vi "prase 4 parameter numeric.vi"(0 "value":string) -> (1 "Settings.Gain.Min 4":dbl, 2 "Settings.Gain.Min 3":dbl, 3 "Settings.Gain.Min 2":dbl, 4 "Settings.Gain.Min":dbl)   [LabVIEW 2011, in "MoveDataFile.lvclass"]
uses:
  MoveDataFile.lvclass
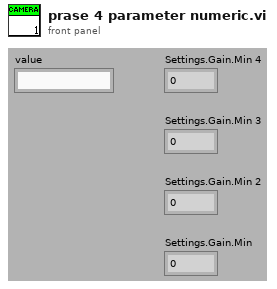
[diagram p1: front panel]
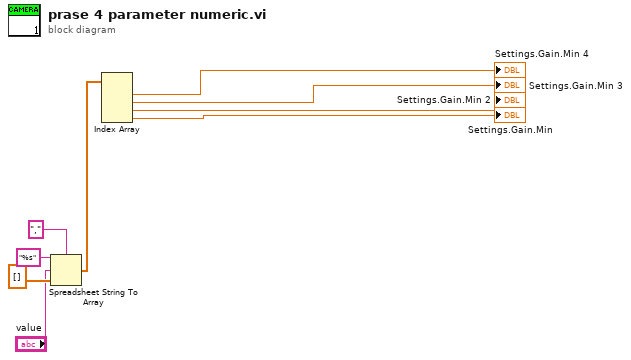
[diagram p0: block diagram]
diagram:
  n1 = Spreadsheet String To Array(delimiter (Tab)=",", format string="%s", spreadsheet string="value", array type (2D Dbl)=dbl[] []) -> (array=w5:dbl[])
  n2 = Index Array(array=w5) -> (element #1=→"Settings.Gain.Min 4":dbl, element #2=→"Settings.Gain.Min 3":dbl, element #3=→"Settings.Gain.Min 2":dbl, element #4=→"Settings.Gain.Min":dbl)  [unwired: 4 in]
